vi "tryRecconect.vi"(8 "error in (no error)":errorcluster, 11 "SharedVariableWrapper in":refnum<class "SharedVariableWrapper.lvclass">) -> (0 "error out":errorcluster)   [LabVIEW 2019, in "SharedVariableWrapper.lvclass"]
uses:
  SharedVariableWrapper.lvclass
  SharedVariableWrapper.lvclass/SharedVariableWrapper.ctl
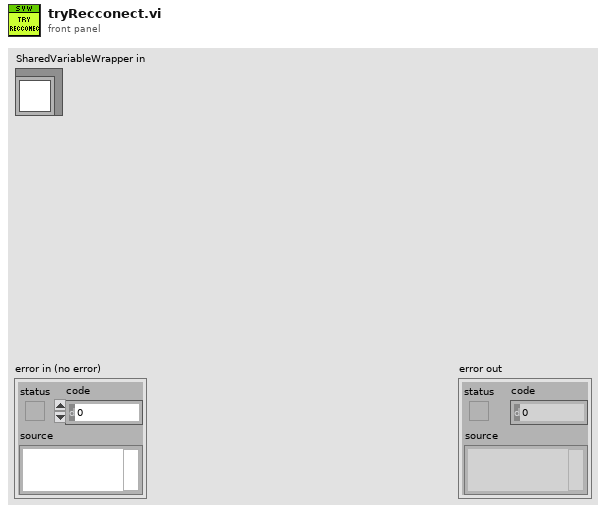
[diagram p1: front panel]
types:
  T1 = typedef "SharedVariableWrapper.lvclass/shared variable info.ctl" = cluster{"shared variable":refnum<k21>, "connected":bool, "Value":variant, "UpdateTime":timestamp}
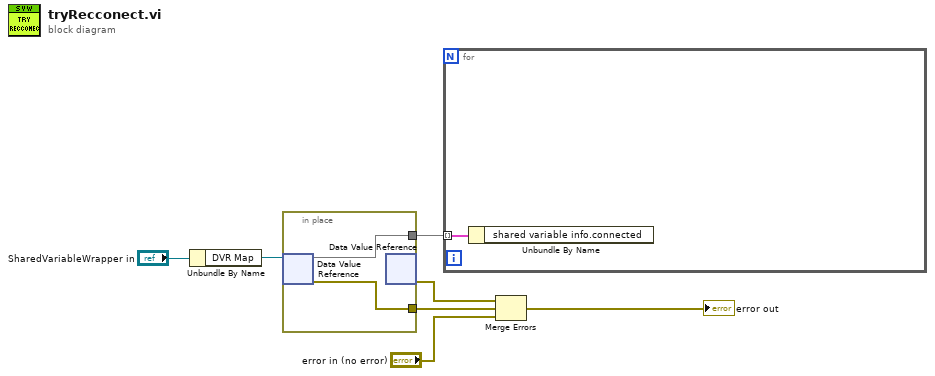
[diagram p0: block diagram]
diagram:
  n1 = Unbundle By Name("SharedVariableWrapper in") -> ("DVR Map"=w5:refnum<data-value>)
  n2 = in-place {
    in-place-border: [w9] -> w2
    in-place-border: [w8] -> w4
    n3 = in-place-dvr #1(w5) -> (w8:map{string, T1}, w9:errorcluster)
    n4 = in-place-dvr #1() -> (w3:errorcluster)  [unwired: 1 in, 1 out]
  }
  n5 = for {
    tunnel: w4 -> [w10] mode=indexing
    n6 = Unbundle By Name(w10) -> ()  [unwired: 1 out]
  }
  n7 = Merge Errors(w3, w2, "error in (no error)") -> (→"error out":errorcluster)
